vi "VariantClusterAccessMulti.vi"(8 "error in (no error)":errorcluster, 9 "labels":string[](array[string]), 10 "indices":i32[](array[numeric]), 11 "Value in":variant) -> (0 "error out":errorcluster, 1 "rest":string, 2 "values":variant[](array[variant]), 3 "prepends":string[](array[string]), 5 "type string":i16[](array[numeric]))   [LabVIEW 2019]
uses:
  <vilib>/Utility/Data Type/NI_Data Type.lvlib
  0df95dc8-5800-4001-9b4d-914d4efa5e44.vi
  b308892c-34a8-450c-8e5e-ad5336504ffd.vi
  83864889-1eb0-4641-a148-0d3fe2e61a46.vi
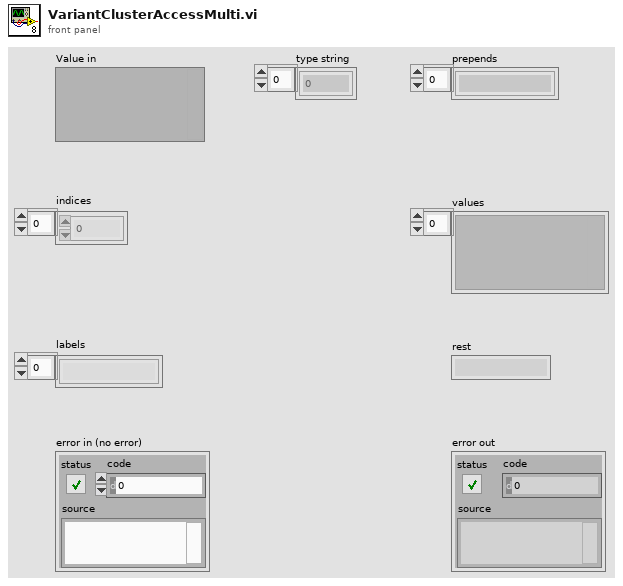
[diagram p1: front panel]
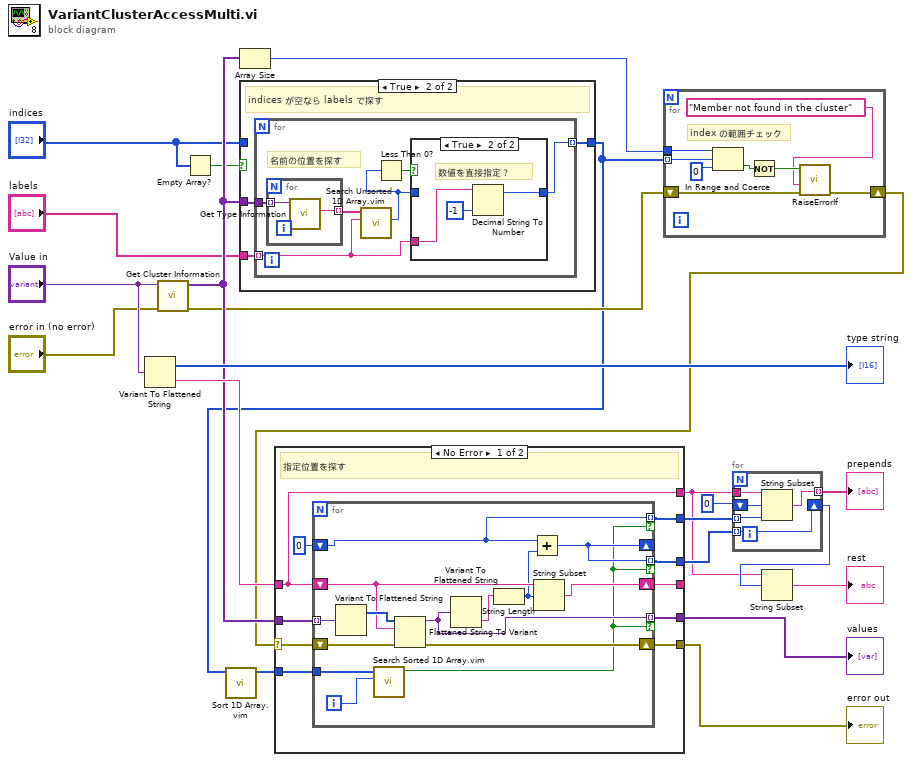
[diagram p0: block diagram]
diagram:
  n1 = Variant To Flattened String(Variant="Value in") -> (data string=w20:string, 1:→"type string":i16[])
  n2 = call <vilib>:"Get Cluster Information.vi"("error in (no error)"="error in (no error)", "variant"="Value in") -> ("error out"=w15:errorcluster, "cluster elements"=w17:variant[])  [unwired: 8 in]
  n3 = Empty Array?(array="indices") -> (empty?=w13:bool)
  n4 = Array Size(array=w17) -> (size(s)=w16:i32)
  n5 = case shown="True" w13 {
    tunnel: w17 -> [_ w26]
    tunnel: "labels" -> [_ w24]
    tunnel: "indices" -> [w23 _]
    tunnel: [w23 w25] -> w11
    frame False {
    }
    frame True {
      # "indices が空なら labels で探す"
      n6 = for {
        tunnel: w26 -> [w32]
        tunnel: [w29] -> w25 mode=indexing
        tunnel: w24 -> [w27] mode=indexing
        # "名前の位置を探す"
        n7 = for {
          tunnel: w32 -> [w38] mode=indexing
          tunnel: [w37] -> w31 mode=indexing
          n8 = call <vilib>:"Get Type Information.vi"("variant"=w38) -> ("name"=w37:string)  [unwired: 6 in, 4 out]
        }
        n9 = call "Search Unsorted 1D Array.vim"("element"=w27, "unsorted 1D array"=w31) -> ("index of element"=w28:i32)  [unwired: 9 in]
        n10 = Less Than 0?(x=w28) -> (x < 0?=w30:bool)
        n11 = case shown="True" w30 {
          tunnel: w27 -> [_ w36]
          tunnel: [w33 w34] -> w29
          tunnel: w28 -> [w33 _]
          frame False {
          }
          frame True {
            # "数値を直接指定？"
            n12 = Decimal String To Number(string=w36, default (0L)=-1 ("default (0 I32)")) -> (offset past number=w34:i32)  [unwired: 1 in, 1 out]
          }
        }
      }
    }
  }
  n13 = call "Sort 1D Array.vim"("unsorted array"=w11) -> ("sorted array"=w1:i32[])  [unwired: 10 in]
  n14 = for {
    tunnel: w16 -> [w46]
    tunnel: w11 -> [w42] mode=indexing
    shift-right: [w40] -> w5
    shift-left: w15 -> [w41]
    # "index の範囲チェック"
    n15 = In Range and Coerce(upper limit=w46, x=w42, lower limit=0) -> (In Range?=w44:bool)  [unwired: 1 out]
    n16 = Not(x=w44) -> (.not. x?=w43:bool)
    n17 = call "RaiseErrorIf.vi"("error in (no error)"=w41, "error message"="Member not found in the cluster", "error? (true)"=w43) -> ("error out"=w40:errorcluster)  [unwired: 8 in]
  }
  n18 = case shown="No Error" w5 {
    selector: w5 -> [w53 w71]
    tunnel: [w56 w71] -> w22
    tunnel: w20 -> [w51 _]
    tunnel: w17 -> [w55 _]
    tunnel: [w52 _] -> w10
    tunnel: [w51 _] -> w3
    tunnel: [w50 _] -> _
    tunnel: [w49 _] -> w6
    tunnel: w1 -> [w48 _]
    tunnel: [w47 _] -> w9
    frame No Error {
      # "指定位置を探す"
      n19 = for {
        tunnel: w55 -> [w65] mode=indexing
        shift-right: [w67] -> w50
        shift-left: w51 -> [w68]
        shift-right: [w64] -> w56
        shift-left: w53 -> [w66]
        shift-right: [w58] -> _
        shift-left: 0 -> [w62]
        tunnel: [w62] -> w52 mode=indexing if=w57
        tunnel: [w61] -> w49 mode=indexing if=w57
        tunnel: w48 -> [w60]
        tunnel: [w58] -> w47 mode=indexing if=w57
        i -> [w59]
        n20 = Variant To Flattened String(Variant=w65) -> (1:w69:i16[])  [unwired: 1 out]
        n21 = call "Search Sorted 1D Array.vim"("element"=w59, "sorted 1D array"=w60) -> ("found?"=w57:bool)  [unwired: 8 in, 1 out]
        n22 = Flattened String To Variant(4:w66, 6:w68, 7:w69) -> (0:w64:errorcluster, 3:w61:variant)
        n23 = Variant To Flattened String(Variant=w61) -> (data string=w70:string)  [unwired: 1 out]
        n24 = String Length(string=w70) -> (length=w63:i32)
        n25 = Add(x=w62, y=w63) -> (x+y=w58:i32)
        n26 = String Subset(string=w68, offset (0)=w63) -> (substring=w67:string)  [unwired: 1 in]
      }
    }
    frame Error {
    }
  }
  "error out" <- w22
  "values" <- w6
  n27 = for {
    tunnel: w3 -> [w75]
    tunnel: w10 -> [w74] mode=indexing
    tunnel: w9 -> [w73] mode=indexing
    shift-right: [w73] -> w4
    shift-left: 0 -> [w76]
    tunnel: [w72] -> w7 mode=indexing
    n28 = String Subset(string=w75, offset (0)=w76, length (rest)=w74) -> (substring=w72:string)
  }
  "prepends" <- w7
  n29 = String Subset(string=w3, offset (0)=w4) -> (substring=→"rest":string)  [unwired: 1 in]
